vi "RSZVB Trace Add S-Parameter Group.vi"(7 "Logical Port Number":i32[](array[numeric]), 8 "error in (no error)":errorcluster {"code" format="%.0x"}, 9 "Number of Logical Port Numbers (1)":i32=1, 10 "Channel (1)":i32=1, 11 "VISA session":refnum<visa-resource-name>) -> (0 "error out":errorcluster {"code" format="%.0x"}, 3 "dup VISA session":refnum<visa-resource-name>)   [LabVIEW 2011]
doc: "This VI creates the traces for all S-parameters associated with a group of logical ports (S-parameter group). \n\nRemote-control command(s):\nCALCulate<Ch>:PARameter:DEFine:SGRoup <log_port1>[, <log_port2>,...]"
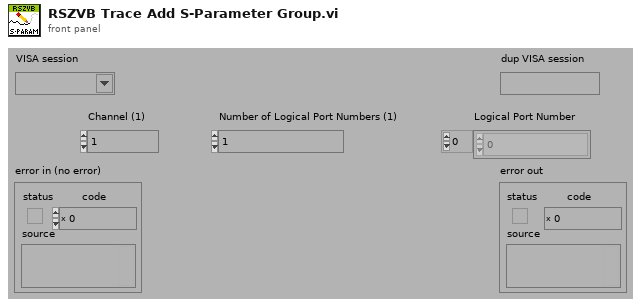
[diagram p1: front panel]
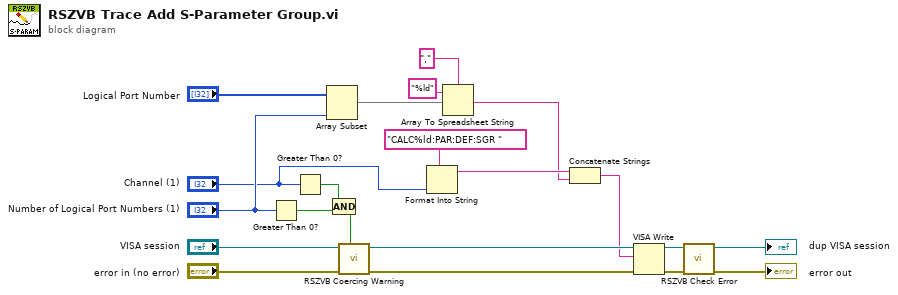
[diagram p0: block diagram]
diagram:
  n1 = Greater Than 0?(x="Number of Logical Port Numbers (1)") -> (x > 0?=w8:bool)
  n2 = Greater Than 0?(x="Channel (1)") -> (x > 0?=w19:bool)
  n3 = Array Subset(array="Logical Port Number", length="Number of Logical Port Numbers (1)") -> (w9:i32[])  [unwired: 1 in]
  n4 = Compound Arithmetic op=AND(w19, w8) -> (w18:bool)
  n5 = call "RSZVB Coercing Warning.vi"("In Range?"=w18, "error in (no error)"="error in (no error)", "VISA session"="VISA session") -> ("error out"=w20:errorcluster, "dup VISA session"=w21:refnum<visa-resource-name>)  [unwired: 7 in]
  n6 = Format Into String(format string="CALC%ld:PAR:DEF:SGR ", "Channel (1)") -> (resulting string=w13:string)  [unwired: 2 in, 1 out]
  n7 = Array To Spreadsheet String(delimiter (Tab)=",", array=w9, 3:"%ld") -> (spreadsheet string=w10:string)
  n8 = Concatenate Strings(w13, w10) -> (w12:string)
  n9 = VISA Write(VISA resource name=w21, write buffer=w12, error in (no error)=w20) -> (VISA resource name out=w15:refnum<visa-resource-name>, error out=w16:errorcluster)  [unwired: 1 out]
  n10 = call "RSZVB Check Error.vi"("error in (no error)"=w16, "VISA session"=w15) -> ("error out"=→"error out":errorcluster, "dup VISA session"=→"dup VISA session":refnum<visa-resource-name>)  [unwired: 8 in]
